vi "File Transfer.vi"(7 "Enum":enum16{"Read", "write"}(ring), 8 "error in":errorcluster, 11 "File transfer in":T1) -> (0 "error out":errorcluster, 3 "File transferout":T1)   [LabVIEW 2022 SP3]
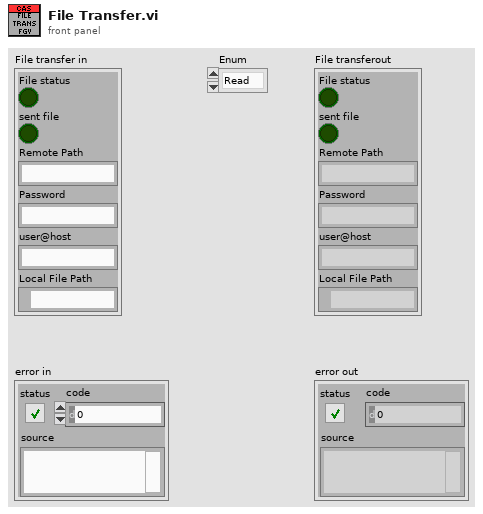
[diagram p1: front panel]
types:
  T1 = cluster{"File status":bool, "sent file":bool, "Remote Path":string, "Password":string, "user@host":string, "Local File Path":path}
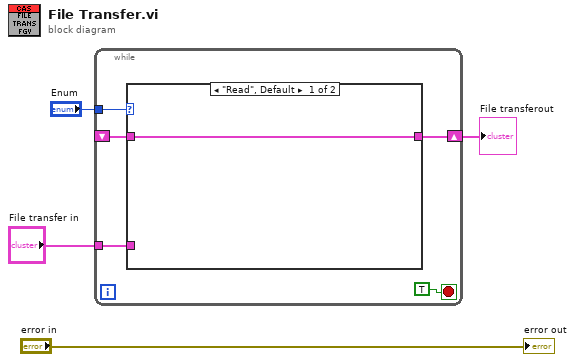
[diagram p0: block diagram]
diagram:
  n1 = while {
    tunnel: "Enum" -> [w8]
    tunnel: "File transfer in" -> [w5]
    shift-right: [w7] -> w2
    shift-left: _ -> [w6]
    stop <- TRUE stop-if-true
    n2 = case shown="\"Read\", Default" w8 {
      tunnel: [w10 w11] -> w7
      tunnel: w6 -> [w10 _]
      tunnel: w5 -> [_ w11]
      frame "Read", Default {
      }
      frame "write" {
      }
    }
  }
  "File transferout" <- w2
  "error out" <- "error in"
